vi "set origin.vi"(8 "error in (no error)":errorcluster, 11 "YK090817SutterMP285Stage in":refnum<class "YK090817SutterMP285Stage.lvclass">=refnum) -> (0 "error out":errorcluster, 3 "YK090817SutterMP285Stage out":refnum<class "YK090817SutterMP285Stage.lvclass">)   [LabVIEW 2010, in "YK090817SutterMP285Stage.lvclass"]
uses:
  YK090817SutterMP285Stage.lvclass
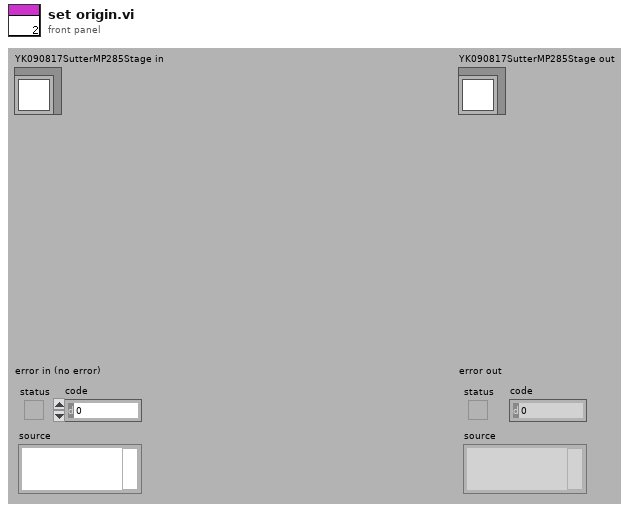
[diagram p1: front panel]
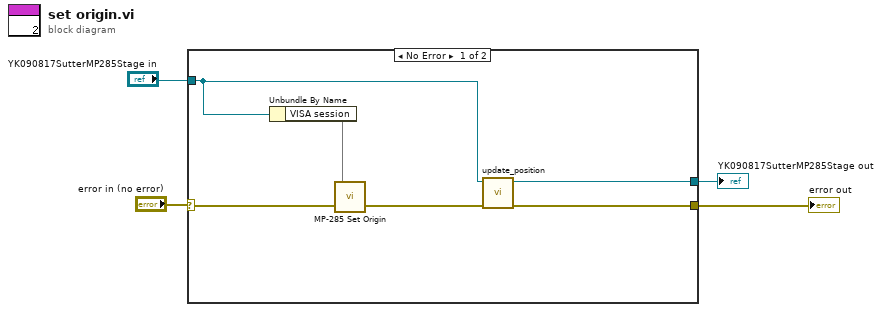
[diagram p0: block diagram]
diagram:
  n1 = case shown="No Error" "error in (no error)" {
    selector: "error in (no error)" -> [w9 w12]
    tunnel: [w7 w12] -> w1
    tunnel: [w5 w11] -> w3
    tunnel: "YK090817SutterMP285Stage in" -> [w6 w11]
    frame No Error {
      n2 = Unbundle By Name(w6) -> ("VISA session"=w10)
      n3 = call "MP-285 Set Origin.vi"("error in (no error)"=w9, "VISA resource name"=w10) -> ("error out"=w8:errorcluster)  [unwired: 1 out]
      n4 = call-dynamic "update_position.vi"("error in (no error)"=w8, "YK090817SutterMP285Stage in"=w6) -> ("error out"=w7:errorcluster, "YK090817SutterMP285Stage out"=w5:refnum<class "YK090817SutterMP285Stage.lvclass">)  [unwired: 8 out]
    }
    frame Error {
    }
  }
  "error out" <- w1
  "YK090817SutterMP285Stage out" <- w3
